vi "Callback - Subscribed names.vi"(8 "error in (no error)":errorcluster, 10 "Subscribed names":string[](array[string]), 11 "BluePlotHandleDemo in":refnum<class "BluePlotHandleDemo.lvclass">) -> (0 "error out":errorcluster, 3 "BluePlotHandleDemo out":refnum<class "BluePlotHandleDemo.lvclass">)   [LabVIEW 2021, in "BluePlotDemo.lvlib" / "BluePlotHandleDemo.lvclass"]
uses:
  BluePlotHandleDemo.lvclass
  BluePlotHandleDemo.lvclass/BluePlotHandleDemo.ctl
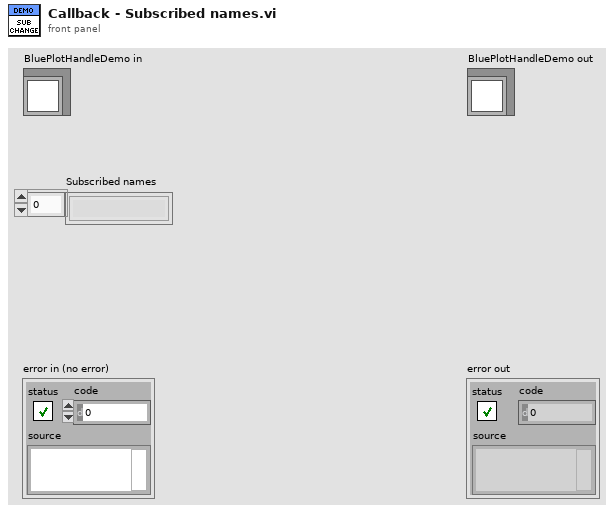
[diagram p1: front panel]
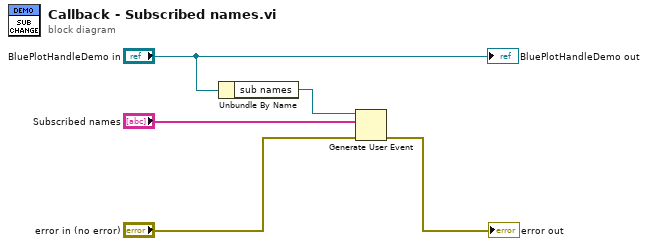
[diagram p0: block diagram]
diagram:
  n1 = Unbundle By Name("BluePlotHandleDemo in") -> ("sub names"=w4:refnum<user-event>)
  n2 = Generate User Event(user event=w4, event data cluster="Subscribed names", error in="error in (no error)") -> (error out=→"error out":errorcluster)  [unwired: 1 in, 1 out]
  "BluePlotHandleDemo out" <- "BluePlotHandleDemo in"
